vi "GetSafetyAndComfortLikerts.vi"(8 "Likert.Results":T1, 10 "Column index in":i32, 11 "Data array in":string[][](array[string])) -> (0 "Likert.Results.out":T1, 3 "Data array out":string[][](array[string]))   [LabVIEW 2025]
uses:
  Controls/Likert.Results.ctl
  Controls/Map.HowSafe.ctl
  Controls/Map.HowComfortable.ctl
  Controls/Map.HowDistracting.ctl
  Controls/Map.HowEasy.ctl
  Controls/Map.EasyBalance.ctl
  Controls/Map.HowPrecisely.ctl
  Controls/Map.HowIntuitive.ctl
  Controls/Map.HowFocussed.ctl
  Controls/Map.LookAway.ctl
  Controls/Map.HowEffortless.ctl
  Controls/Map.HowConfident.ctl
  Controls/Map.DontInterfere.ctl
  Controls/Map.Enjoyment.ctl
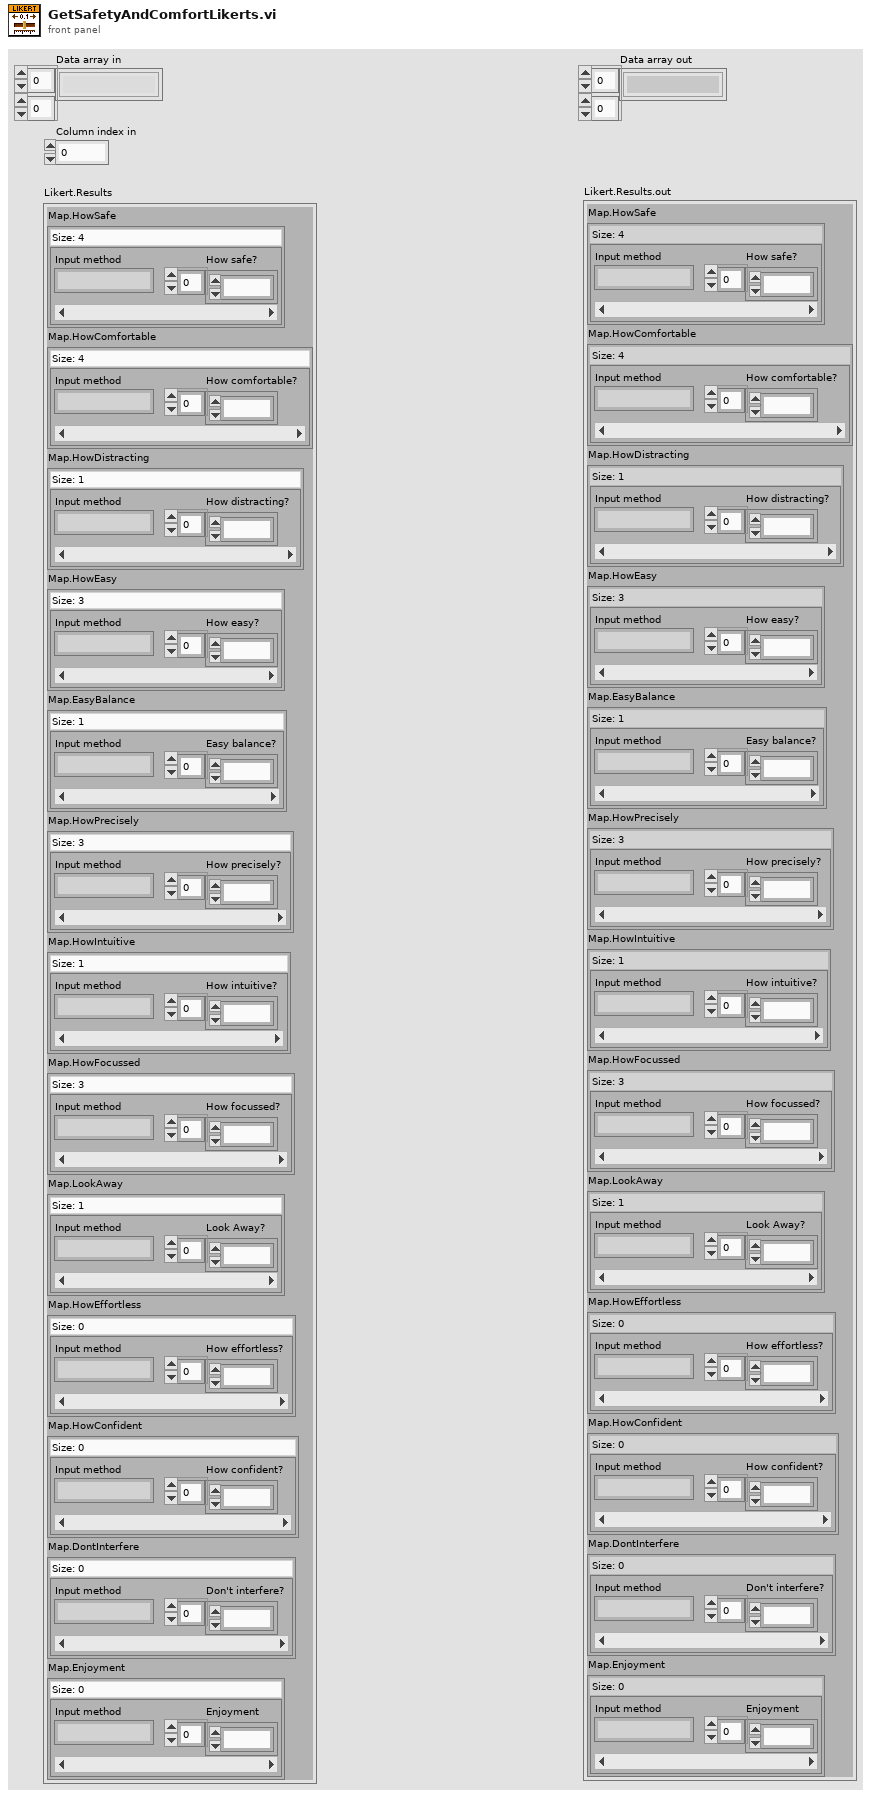
[diagram p1: front panel]
types:
  T1 = typedef "Likert.Results.ctl" = cluster{"Map.HowSafe":T2, "Map.HowComfortable":T3, "Map.HowDistracting":T4, "Map.HowEasy":T5, "Map.EasyBalance":T6, "Map.HowPrecisely":T7, "Map.HowIntuitive":T8, "Map.HowFocussed":T9, "Map.LookAway":T10, "Map.HowEffortless":T11, "Map.HowConfident":T12, "Map.DontInterfere":T13, "Map.Enjoyment":T14}
  T2 = typedef "Map.HowSafe.ctl" = map{string, i32[]}
  T3 = typedef "Map.HowComfortable.ctl" = map{string, i32[]}
  T4 = typedef "Map.HowDistracting.ctl" = map{string, i32[]}
  T5 = typedef "Map.HowEasy.ctl" = map{string, i32[]}
  T6 = typedef "Map.EasyBalance.ctl" = map{string, i32[]}
  T7 = typedef "Map.HowPrecisely.ctl" = map{string, i32[]}
  T8 = typedef "Map.HowIntuitive.ctl" = map{string, i32[]}
  T9 = typedef "Map.HowFocussed.ctl" = map{string, i32[]}
  T10 = typedef "Map.LookAway.ctl" = map{string, i32[]}
  T11 = typedef "Map.HowEffortless.ctl" = map{string, i32[]}
  T12 = typedef "Map.HowConfident.ctl" = map{string, i32[]}
  T13 = typedef "Map.DontInterfere.ctl" = map{string, i32[]}
  T14 = typedef "Map.Enjoyment.ctl" = map{string, i32[]}
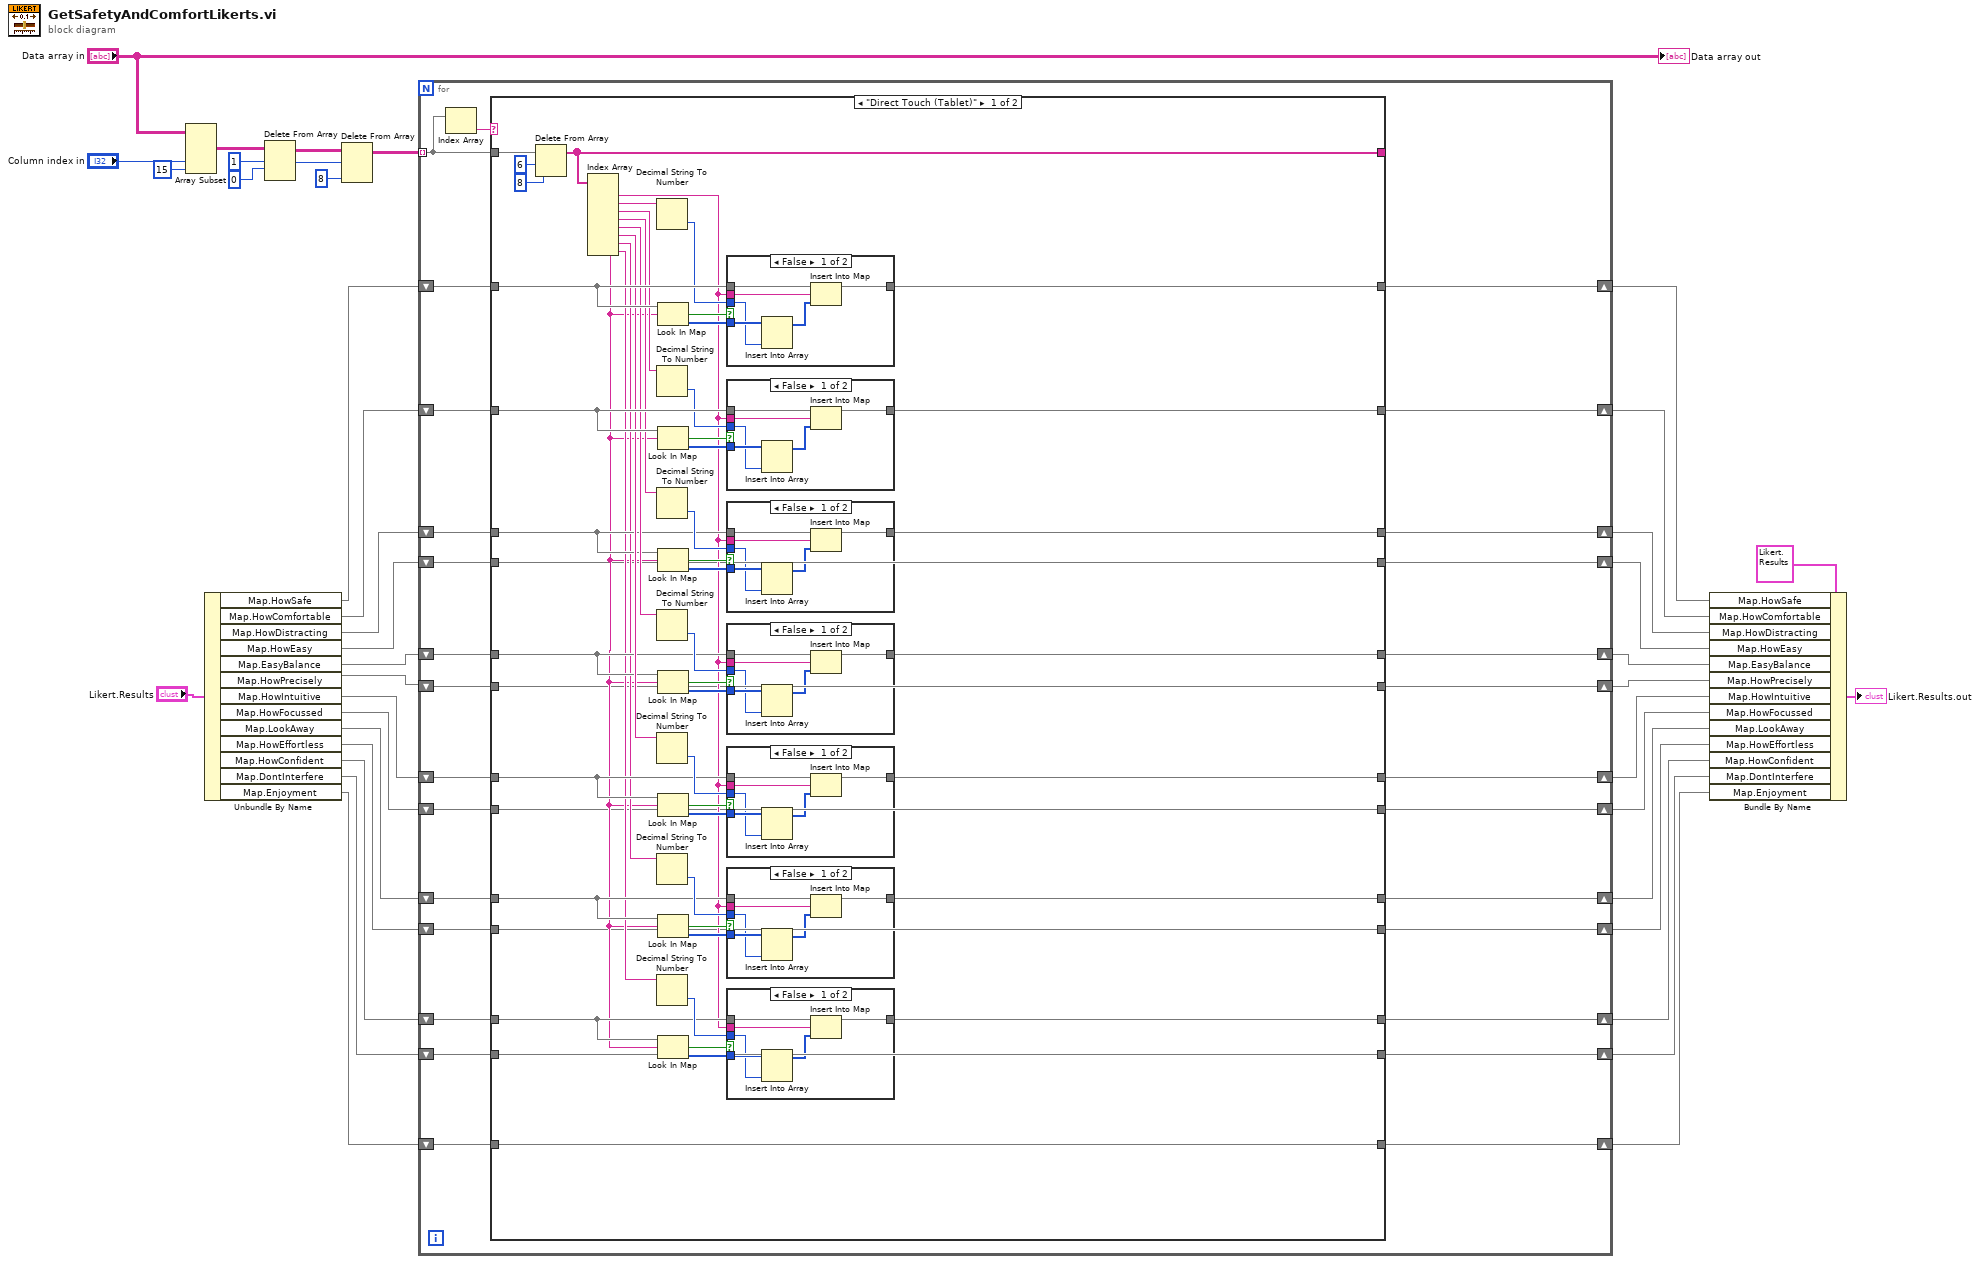
[diagram p0: block diagram]
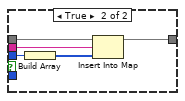
[diagram p2: hidden frame]
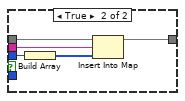
[diagram p3: hidden frame]
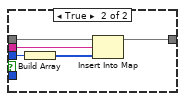
[diagram p4: hidden frame]
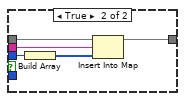
[diagram p5: hidden frame]
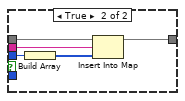
[diagram p6: hidden frame]
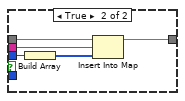
[diagram p7: hidden frame]
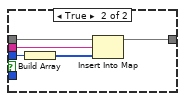
[diagram p8: hidden frame]
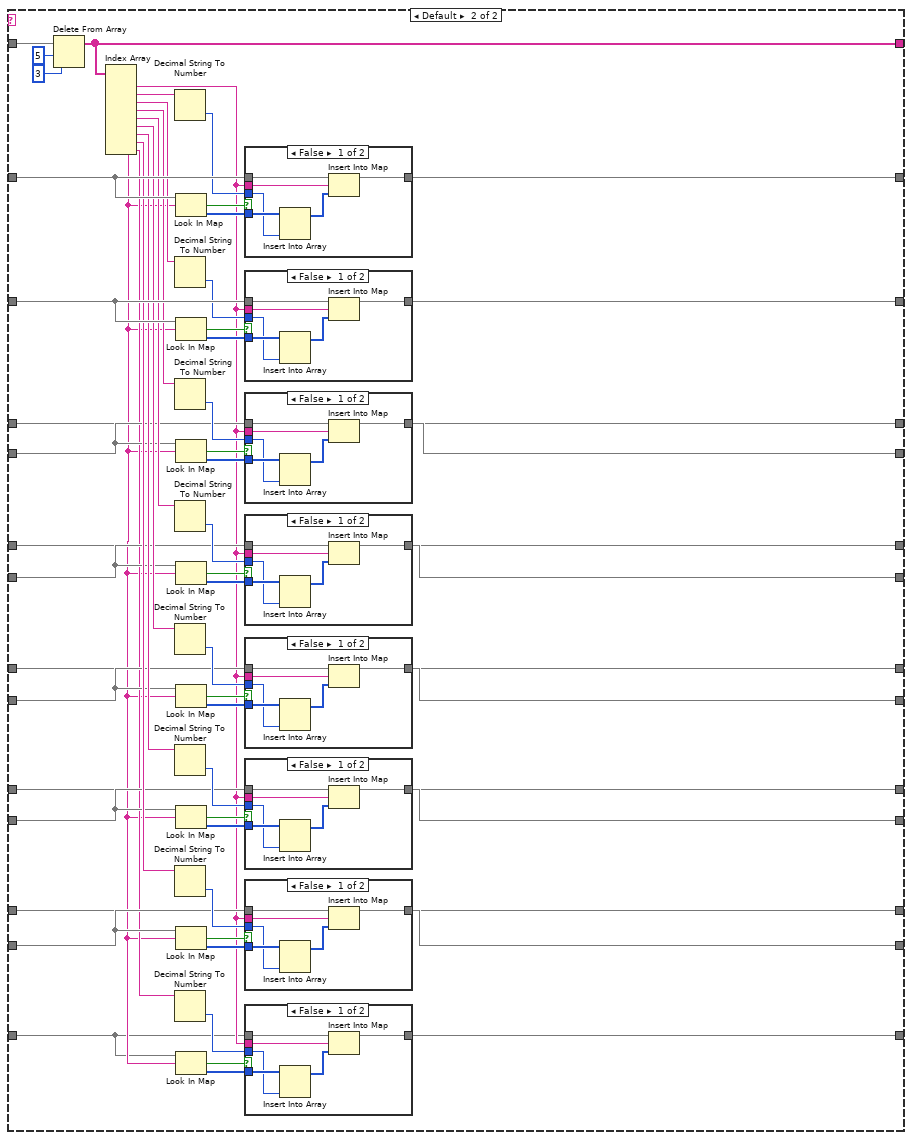
[diagram p9: hidden frame]
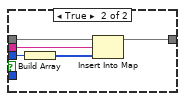
[diagram p10: hidden frame]
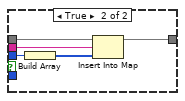
[diagram p11: hidden frame]
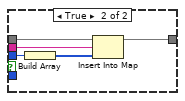
[diagram p12: hidden frame]
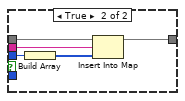
[diagram p13: hidden frame]
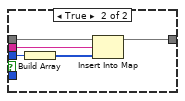
[diagram p14: hidden frame]
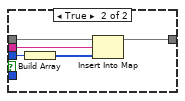
[diagram p15: hidden frame]
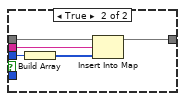
[diagram p16: hidden frame]
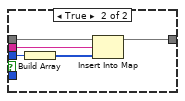
[diagram p17: hidden frame]
diagram:
  w33 = 1 ("length")
  n1 = Array Subset(array="Data array in", index (col)="Column index in", length (col)=15 ("length")) -> (w31:string[][])  [unwired: 2 in]
  n2 = Unbundle By Name("Likert.Results") -> ("Map.HowSafe"=w28:T2, "Map.HowComfortable"=w27:T3, "Map.HowDistracting"=w26:T4, "Map.HowEasy"=w25:T5, "Map.EasyBalance"=w24:T6, "Map.HowPrecisely"=w23:T7, "Map.HowIntuitive"=w22:T8, "Map.HowFocussed"=w21:T9, "Map.LookAway"=w20:T10, "Map.HowEffortless"=w19:T11, "Map.HowConfident"=w18:T12, "Map.DontInterfere"=w17:T13, "Map.Enjoyment"=w16:T14)
  n3 = Delete From Array(array=w31, length=w33, index (row)=0) -> (array with subset deleted=w34:string[][])  [unwired: 1 in, 1 out]
  n4 = Delete From Array(array=w34, length=w33, index (col)=8 ("disabled index (col)")) -> (array with subset deleted=w30:string[][])  [unwired: 1 in, 1 out]
  n5 = for {
    tunnel: w30 -> [w65] mode=indexing
    shift-right: [w63] -> w14
    shift-left: w28 -> [w64]
    shift-right: [w61] -> w13
    shift-left: w27 -> [w62]
    shift-right: [w59] -> w12
    shift-left: w26 -> [w60]
    shift-right: [w57] -> w10
    shift-left: w24 -> [w58]
    shift-right: [w55] -> w8
    shift-left: w22 -> [w56]
    shift-right: [w52] -> w6
    shift-left: w20 -> [w54]
    shift-right: [w51] -> w4
    shift-left: w18 -> [w53]
    shift-right: [w49] -> w11
    shift-left: w25 -> [w50]
    shift-right: [w47] -> w9
    shift-left: w23 -> [w48]
    shift-right: [w45] -> w7
    shift-left: w21 -> [w46]
    shift-right: [w43] -> w5
    shift-left: w19 -> [w44]
    shift-right: [w41] -> w3
    shift-left: w17 -> [w42]
    shift-right: [w39] -> w2
    shift-left: w16 -> [w40]
    n6 = Index Array(array=w65) -> (element=w66:string)  [unwired: 1 in]
    n7 = case shown="\"Direct Touch (Tablet)\"" w66 {
      tunnel: w65 -> [w119 w254]
      tunnel: [w116 w251] -> _
      tunnel: w64 -> [w113 w248]
      tunnel: [w114 w249] -> w63
      tunnel: w62 -> [w106 w241]
      tunnel: [w108 w243] -> w61
      tunnel: w60 -> [w89 w216]
      tunnel: [w94 w216] -> w59
      tunnel: w58 -> [w88 w213]
      tunnel: [w93 w213] -> w57
      tunnel: w56 -> [w87 w210]
      tunnel: [w86 w210] -> w55
      tunnel: w54 -> [w78 w207]
      tunnel: w53 -> [w76 w204]
      tunnel: [w74 w207] -> w52
      tunnel: [w73 w204] -> w51
      tunnel: w50 -> [w72 w218]
      tunnel: [w72 w217] -> w49
      tunnel: w48 -> [w71 w215]
      tunnel: [w71 w214] -> w47
      tunnel: w46 -> [w70 w212]
      tunnel: [w70 w211] -> w45
      tunnel: w44 -> [w69 w209]
      tunnel: [w69 w208] -> w43
      tunnel: w42 -> [w68 w206]
      tunnel: [w68 w205] -> w41
      tunnel: w40 -> [w67 w197]
      tunnel: [w67 w200] -> w39
      frame "Direct Touch (Tablet)" {
        n8 = Delete From Array(array=w119, length=6, index=8) -> (array with subset deleted=w116:string[])  [unwired: 1 out]
        n9 = Index Array(array=w116) -> (element #1=w75:string, element #2=w112:string, element #3=w107:string, element #4=w92:string, element #5=w91:string, element #6=w90:string, element #7=w79:string, element #8=w77:string)  [unwired: 8 in]
        n10 = Decimal String To Number(string=w112) -> (number=w105:i32)  [unwired: 2 in, 1 out]
        n11 = Decimal String To Number(string=w107) -> (number=w104:i32)  [unwired: 2 in, 1 out]
        n12 = Decimal String To Number(string=w92) -> (number=w103:i32)  [unwired: 2 in, 1 out]
        n13 = Decimal String To Number(string=w91) -> (number=w98:i32)  [unwired: 2 in, 1 out]
        n14 = Decimal String To Number(string=w90) -> (number=w97:i32)  [unwired: 2 in, 1 out]
        n15 = Decimal String To Number(string=w79) -> (number=w83:i32)  [unwired: 2 in, 1 out]
        n16 = Decimal String To Number(string=w77) -> (number=w82:i32)  [unwired: 2 in, 1 out]
        n17 = Look In Map(map=w113, key=w75) -> (key not found?=w115:bool, value=w111:i32[])  [unwired: 1 in]
        n18 = Look In Map(map=w106, key=w75) -> (key not found?=w109:bool, value=w110:i32[])  [unwired: 1 in]
        n19 = Look In Map(map=w89, key=w75) -> (key not found?=w102:bool, value=w101:i32[])  [unwired: 1 in]
        n20 = Look In Map(map=w88, key=w75) -> (key not found?=w99:bool, value=w100:i32[])  [unwired: 1 in]
        n21 = Look In Map(map=w87, key=w75) -> (key not found?=w96:bool, value=w95:i32[])  [unwired: 1 in]
        n22 = Look In Map(map=w78, key=w75) -> (key not found?=w84:bool, value=w85:i32[])  [unwired: 1 in]
        n23 = Look In Map(map=w76, key=w75) -> (key not found?=w81:bool, value=w80:i32[])  [unwired: 1 in]
        n24 = case shown="False" w115 {
          tunnel: w113 -> [w191 w196]
          tunnel: [w190 w195] -> w114
          tunnel: w75 -> [w189 w194]
          tunnel: w105 -> [w187 w193]
          tunnel: w111 -> [w188 _]
          frame False {
            n25 = Insert Into Array(array=w188, new element=w187) -> (w186:i32[])  [unwired: 1 in]
            n26 = Insert Into Map(map in=w191, key=w189, value=w186) -> (map out=w190:T2)  [unwired: 2 out]
          }
          frame True {
            n27 = Build Array(w193) -> (w192:i32[])
            n28 = Insert Into Map(map in=w196, key=w194, value=w192) -> (map out=w195:T2)  [unwired: 2 out]
          }
        }
        n29 = case shown="False" w109 {
          tunnel: w106 -> [w180 w185]
          tunnel: [w179 w184] -> w108
          tunnel: w75 -> [w178 w183]
          tunnel: w104 -> [w176 w182]
          tunnel: w110 -> [w177 _]
          frame False {
            n30 = Insert Into Array(array=w177, new element=w176) -> (w175:i32[])  [unwired: 1 in]
            n31 = Insert Into Map(map in=w180, key=w178, value=w175) -> (map out=w179:T3)  [unwired: 2 out]
          }
          frame True {
            n32 = Build Array(w182) -> (w181:i32[])
            n33 = Insert Into Map(map in=w185, key=w183, value=w181) -> (map out=w184:T3)  [unwired: 2 out]
          }
        }
        n34 = case shown="False" w102 {
          tunnel: w89 -> [w169 w174]
          tunnel: [w168 w173] -> w94
          tunnel: w75 -> [w167 w172]
          tunnel: w103 -> [w165 w171]
          tunnel: w101 -> [w166 _]
          frame False {
            n35 = Insert Into Array(array=w166, new element=w165) -> (w164:i32[])  [unwired: 1 in]
            n36 = Insert Into Map(map in=w169, key=w167, value=w164) -> (map out=w168:T4)  [unwired: 2 out]
          }
          frame True {
            n37 = Build Array(w171) -> (w170:i32[])
            n38 = Insert Into Map(map in=w174, key=w172, value=w170) -> (map out=w173:T4)  [unwired: 2 out]
          }
        }
        n39 = case shown="False" w99 {
          tunnel: w88 -> [w158 w163]
          tunnel: [w157 w162] -> w93
          tunnel: w75 -> [w156 w161]
          tunnel: w98 -> [w154 w160]
          tunnel: w100 -> [w155 _]
          frame False {
            n40 = Insert Into Array(array=w155, new element=w154) -> (w153:i32[])  [unwired: 1 in]
            n41 = Insert Into Map(map in=w158, key=w156, value=w153) -> (map out=w157:T6)  [unwired: 2 out]
          }
          frame True {
            n42 = Build Array(w160) -> (w159:i32[])
            n43 = Insert Into Map(map in=w163, key=w161, value=w159) -> (map out=w162:T6)  [unwired: 2 out]
          }
        }
        n44 = case shown="False" w96 {
          tunnel: w87 -> [w147 w152]
          tunnel: [w146 w151] -> w86
          tunnel: w75 -> [w145 w150]
          tunnel: w97 -> [w143 w149]
          tunnel: w95 -> [w144 _]
          frame False {
            n45 = Insert Into Array(array=w144, new element=w143) -> (w142:i32[])  [unwired: 1 in]
            n46 = Insert Into Map(map in=w147, key=w145, value=w142) -> (map out=w146:T8)  [unwired: 2 out]
          }
          frame True {
            n47 = Build Array(w149) -> (w148:i32[])
            n48 = Insert Into Map(map in=w152, key=w150, value=w148) -> (map out=w151:T8)  [unwired: 2 out]
          }
        }
        n49 = case shown="False" w84 {
          tunnel: w78 -> [w136 w141]
          tunnel: [w135 w140] -> w74
          tunnel: w75 -> [w134 w139]
          tunnel: w83 -> [w132 w138]
          tunnel: w85 -> [w133 _]
          frame False {
            n50 = Insert Into Array(array=w133, new element=w132) -> (w131:i32[])  [unwired: 1 in]
            n51 = Insert Into Map(map in=w136, key=w134, value=w131) -> (map out=w135:T10)  [unwired: 2 out]
          }
          frame True {
            n52 = Build Array(w138) -> (w137:i32[])
            n53 = Insert Into Map(map in=w141, key=w139, value=w137) -> (map out=w140:T10)  [unwired: 2 out]
          }
        }
        n54 = case shown="False" w81 {
          tunnel: w76 -> [w125 w130]
          tunnel: [w124 w129] -> w73
          tunnel: w75 -> [w123 w128]
          tunnel: w82 -> [w121 w127]
          tunnel: w80 -> [w122 _]
          frame False {
            n55 = Insert Into Array(array=w122, new element=w121) -> (w120:i32[])  [unwired: 1 in]
            n56 = Insert Into Map(map in=w125, key=w123, value=w120) -> (map out=w124:T12)  [unwired: 2 out]
          }
          frame True {
            n57 = Build Array(w127) -> (w126:i32[])
            n58 = Insert Into Map(map in=w130, key=w128, value=w126) -> (map out=w129:T12)  [unwired: 2 out]
          }
        }
      }
      frame Default {
        n59 = Delete From Array(array=w254, length=5, index=3) -> (array with subset deleted=w251:string[])  [unwired: 1 out]
        n60 = Index Array(array=w251) -> (element #1=w198:string, element #2=w247:string, element #3=w242:string, element #4=w229:string, element #5=w228:string, element #6=w227:string, element #7=w220:string, element #8=w219:string, element #9=w199:string)  [unwired: 9 in]
        n61 = Decimal String To Number(string=w247) -> (number=w240:i32)  [unwired: 2 in, 1 out]
        n62 = Decimal String To Number(string=w242) -> (number=w239:i32)  [unwired: 2 in, 1 out]
        n63 = Decimal String To Number(string=w229) -> (number=w238:i32)  [unwired: 2 in, 1 out]
        n64 = Decimal String To Number(string=w228) -> (number=w233:i32)  [unwired: 2 in, 1 out]
        n65 = Decimal String To Number(string=w227) -> (number=w232:i32)  [unwired: 2 in, 1 out]
        n66 = Decimal String To Number(string=w220) -> (number=w224:i32)  [unwired: 2 in, 1 out]
        n67 = Decimal String To Number(string=w219) -> (number=w223:i32)  [unwired: 2 in, 1 out]
        n68 = Decimal String To Number(string=w199) -> (number=w201:i32)  [unwired: 2 in, 1 out]
        n69 = Look In Map(map=w248, key=w198) -> (key not found?=w250:bool, value=w246:i32[])  [unwired: 1 in]
        n70 = Look In Map(map=w241, key=w198) -> (key not found?=w244:bool, value=w245:i32[])  [unwired: 1 in]
        n71 = Look In Map(map=w218, key=w198) -> (key not found?=w237:bool, value=w236:i32[])  [unwired: 1 in]
        n72 = Look In Map(map=w215, key=w198) -> (key not found?=w234:bool, value=w235:i32[])  [unwired: 1 in]
        n73 = Look In Map(map=w212, key=w198) -> (key not found?=w231:bool, value=w230:i32[])  [unwired: 1 in]
        n74 = Look In Map(map=w209, key=w198) -> (key not found?=w225:bool, value=w226:i32[])  [unwired: 1 in]
        n75 = Look In Map(map=w206, key=w198) -> (key not found?=w222:bool, value=w221:i32[])  [unwired: 1 in]
        n76 = Look In Map(map=w197, key=w198) -> (key not found?=w202:bool, value=w203:i32[])  [unwired: 1 in]
        n77 = case shown="False" w250 {
          tunnel: w248 -> [w337 w342]
          tunnel: [w336 w341] -> w249
          tunnel: w198 -> [w335 w340]
          tunnel: w240 -> [w333 w339]
          tunnel: w246 -> [w334 _]
          frame False {
            n78 = Insert Into Array(array=w334, new element=w333) -> (w332:i32[])  [unwired: 1 in]
            n79 = Insert Into Map(map in=w337, key=w335, value=w332) -> (map out=w336:T2)  [unwired: 2 out]
          }
          frame True {
            n80 = Build Array(w339) -> (w338:i32[])
            n81 = Insert Into Map(map in=w342, key=w340, value=w338) -> (map out=w341:T2)  [unwired: 2 out]
          }
        }
        n82 = case shown="False" w244 {
          tunnel: w241 -> [w326 w331]
          tunnel: [w325 w330] -> w243
          tunnel: w198 -> [w324 w329]
          tunnel: w239 -> [w322 w328]
          tunnel: w245 -> [w323 _]
          frame False {
            n83 = Insert Into Array(array=w323, new element=w322) -> (w321:i32[])  [unwired: 1 in]
            n84 = Insert Into Map(map in=w326, key=w324, value=w321) -> (map out=w325:T3)  [unwired: 2 out]
          }
          frame True {
            n85 = Build Array(w328) -> (w327:i32[])
            n86 = Insert Into Map(map in=w331, key=w329, value=w327) -> (map out=w330:T3)  [unwired: 2 out]
          }
        }
        n87 = case shown="False" w237 {
          tunnel: w218 -> [w315 w320]
          tunnel: [w314 w319] -> w217
          tunnel: w198 -> [w313 w318]
          tunnel: w238 -> [w311 w317]
          tunnel: w236 -> [w312 _]
          frame False {
            n88 = Insert Into Array(array=w312, new element=w311) -> (w310:i32[])  [unwired: 1 in]
            n89 = Insert Into Map(map in=w315, key=w313, value=w310) -> (map out=w314:T5)  [unwired: 2 out]
          }
          frame True {
            n90 = Build Array(w317) -> (w316:i32[])
            n91 = Insert Into Map(map in=w320, key=w318, value=w316) -> (map out=w319:T5)  [unwired: 2 out]
          }
        }
        n92 = case shown="False" w234 {
          tunnel: w215 -> [w304 w309]
          tunnel: [w303 w308] -> w214
          tunnel: w198 -> [w302 w307]
          tunnel: w233 -> [w300 w306]
          tunnel: w235 -> [w301 _]
          frame False {
            n93 = Insert Into Array(array=w301, new element=w300) -> (w299:i32[])  [unwired: 1 in]
            n94 = Insert Into Map(map in=w304, key=w302, value=w299) -> (map out=w303:T7)  [unwired: 2 out]
          }
          frame True {
            n95 = Build Array(w306) -> (w305:i32[])
            n96 = Insert Into Map(map in=w309, key=w307, value=w305) -> (map out=w308:T7)  [unwired: 2 out]
          }
        }
        n97 = case shown="False" w231 {
          tunnel: w212 -> [w293 w298]
          tunnel: [w292 w297] -> w211
          tunnel: w198 -> [w291 w296]
          tunnel: w232 -> [w289 w295]
          tunnel: w230 -> [w290 _]
          frame False {
            n98 = Insert Into Array(array=w290, new element=w289) -> (w288:i32[])  [unwired: 1 in]
            n99 = Insert Into Map(map in=w293, key=w291, value=w288) -> (map out=w292:T9)  [unwired: 2 out]
          }
          frame True {
            n100 = Build Array(w295) -> (w294:i32[])
            n101 = Insert Into Map(map in=w298, key=w296, value=w294) -> (map out=w297:T9)  [unwired: 2 out]
          }
        }
        n102 = case shown="False" w225 {
          tunnel: w209 -> [w282 w287]
          tunnel: [w281 w286] -> w208
          tunnel: w198 -> [w280 w285]
          tunnel: w224 -> [w278 w284]
          tunnel: w226 -> [w279 _]
          frame False {
            n103 = Insert Into Array(array=w279, new element=w278) -> (w277:i32[])  [unwired: 1 in]
            n104 = Insert Into Map(map in=w282, key=w280, value=w277) -> (map out=w281:T11)  [unwired: 2 out]
          }
          frame True {
            n105 = Build Array(w284) -> (w283:i32[])
            n106 = Insert Into Map(map in=w287, key=w285, value=w283) -> (map out=w286:T11)  [unwired: 2 out]
          }
        }
        n107 = case shown="False" w222 {
          tunnel: w206 -> [w271 w276]
          tunnel: [w270 w275] -> w205
          tunnel: w198 -> [w269 w274]
          tunnel: w223 -> [w267 w273]
          tunnel: w221 -> [w268 _]
          frame False {
            n108 = Insert Into Array(array=w268, new element=w267) -> (w266:i32[])  [unwired: 1 in]
            n109 = Insert Into Map(map in=w271, key=w269, value=w266) -> (map out=w270:T13)  [unwired: 2 out]
          }
          frame True {
            n110 = Build Array(w273) -> (w272:i32[])
            n111 = Insert Into Map(map in=w276, key=w274, value=w272) -> (map out=w275:T13)  [unwired: 2 out]
          }
        }
        n112 = case shown="False" w202 {
          tunnel: w197 -> [w260 w265]
          tunnel: [w259 w264] -> w200
          tunnel: w198 -> [w258 w263]
          tunnel: w201 -> [w256 w262]
          tunnel: w203 -> [w257 _]
          frame False {
            n113 = Insert Into Array(array=w257, new element=w256) -> (w255:i32[])  [unwired: 1 in]
            n114 = Insert Into Map(map in=w260, key=w258, value=w255) -> (map out=w259:T14)  [unwired: 2 out]
          }
          frame True {
            n115 = Build Array(w262) -> (w261:i32[])
            n116 = Insert Into Map(map in=w265, key=w263, value=w261) -> (map out=w264:T14)  [unwired: 2 out]
          }
        }
      }
    }
  }
  n117 = Bundle By Name(cluster=T1 {"Map.HowSafe"={}, "Map.HowComfortable"={}, "Map.HowDistracting"={}, "Map.HowEasy"={}, "Map.EasyBalance"={}, "Map.HowPrecisely"={}, "Map.HowIntuitive"={}, "Map.HowFocussed"={}, "Map.LookAway"={}, "Map.HowEffortless"={}, "Map.HowConfident"={}, "Map.DontInterfere"={}, "Map.Enjoyment"={}} ("Likert.Results"), "Map.HowSafe"=w14, "Map.HowComfortable"=w13, "Map.HowDistracting"=w12, "Map.HowEasy"=w11, "Map.EasyBalance"=w10, "Map.HowPrecisely"=w9, "Map.HowIntuitive"=w8, "Map.HowFocussed"=w7, "Map.LookAway"=w6, "Map.HowEffortless"=w5, "Map.HowConfident"=w4, "Map.DontInterfere"=w3, "Map.Enjoyment"=w2) -> (→"Likert.Results.out":T1)
  "Data array out" <- "Data array in"
